vi "Get Calibration Data.vi"(0 "Base Path":path, 2 "Test Type":T1=1 items=["Practice Trials", "Mechanical (Mask)", "Mechanical (Mouthpiece)", "Labial (Normal)", "Labial (Quiet)", "Incomplete Interrupter", "Airflow Redirector", "Singing Helmet"], 5 "error in (no error)":errorcluster) -> (14 "Pressure Slope":dbl, 15 "Pressure Intercept":dbl, 16 "Microphone Sensitivity":dbl, 17 "SPL Gain":dbl, 18 "Flow Array":dbl[](array[numeric]), 19 "error out":errorcluster)   [LabVIEW 2020]
uses:
  Controls/Mech-Labial Test Types.ctl
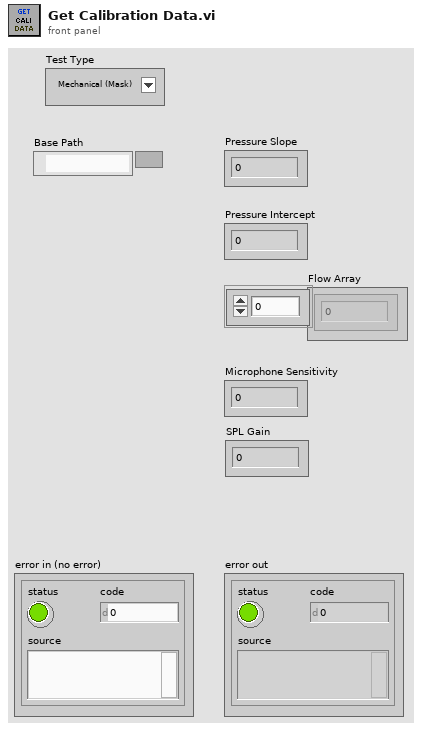
[diagram p1: front panel]
types:
  T1 = typedef "Mech-Labial Test Types.ctl" = u16
  T2 = enum16{"open", "replace", "create", "open or create", "replace or create", "replace or create with confirmation"}
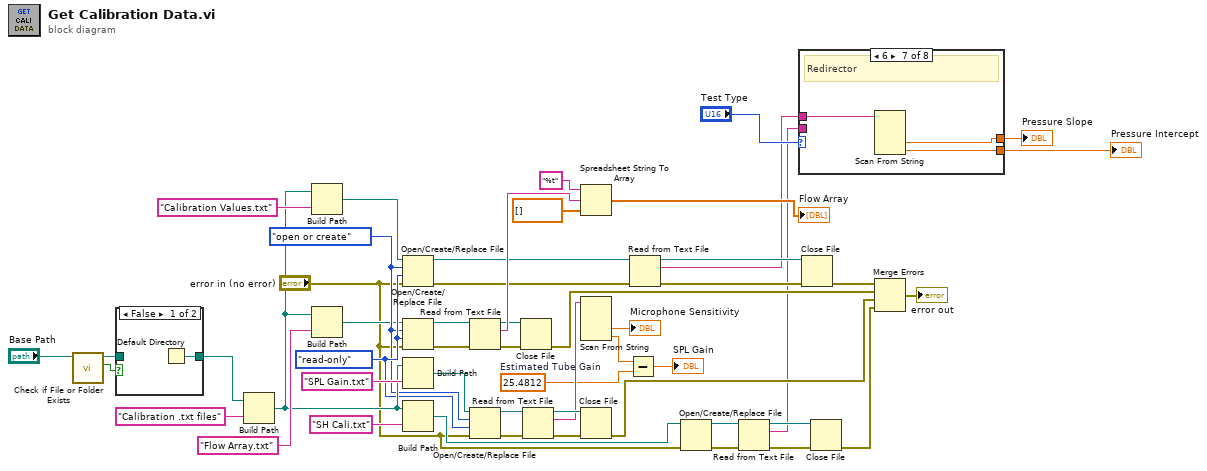
[diagram p0: block diagram]
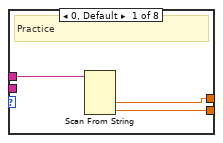
[diagram p2: hidden frame]
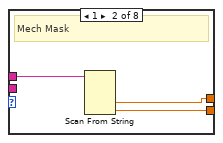
[diagram p3: hidden frame]
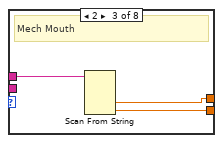
[diagram p4: hidden frame]
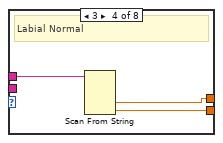
[diagram p5: hidden frame]
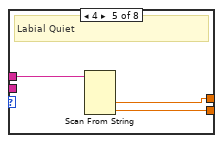
[diagram p6: hidden frame]
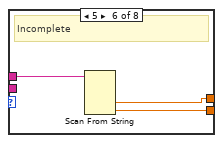
[diagram p7: hidden frame]
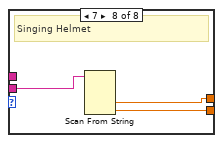
[diagram p8: hidden frame]
diagram:
  w6 = 25.4812  # Estimated Tube Gain
  w36 = enum16{"read/write", "read-only", "write-only"}."read-only" ("access (0:read/write)")
  w35 = T2."open or create" ("operation (0:open)")
  n1 = call <vilib>:"Check if File or Folder Exists.vi"("path"="Base Path") -> ("file or folder exists?"=w47:bool, "dup path"=w46:path)  [unwired: 8 in, 1 out]
  n2 = case shown="False" w47 {
    tunnel: w46 -> [_ w54]
    tunnel: [w53 w54] -> w45
    frame False {
      n3 = Default Directory() -> (w53:path)
    }
    frame True {
    }
  }
  n4 = Build Path(base path=w45, name or relative path="Calibration .txt files") -> (appended path=w44:path)
  n5 = Build Path(base path=w44, name or relative path="Calibration Values.txt") -> (appended path=w15:path)
  n6 = Build Path(base path=w44, name or relative path="Flow Array.txt") -> (appended path=w16:path)
  n7 = Open/Create/Replace File(file path (use dialog)=w15, error in="error in (no error)", operation (0:open)=w35, access (0:read/write)=w36) -> (refnum out=w19:refnum<file>, error out=w17:errorcluster)  [unwired: 2 in, 1 out]
  n8 = Open/Create/Replace File(file path (use dialog)=w16, error in="error in (no error)", operation (0:open)=w35, access (0:read/write)=w36) -> (refnum out=w23:refnum<file>, error out=w21:errorcluster)  [unwired: 2 in, 1 out]
  n9 = Build Path(base path=w44, name or relative path="SPL Gain.txt") -> (appended path=w14:path)
  n10 = Build Path(base path=w44, name or relative path="SH Cali.txt") -> (appended path=w13:path)
  n11 = Read from Text File(file (use dialog)=w23, error in=w21) -> (refnum out=w24:refnum<file>, text=w29:string, error out=w22:errorcluster)  [unwired: 2 in, 1 out]
  n12 = Open/Create/Replace File(file path (use dialog)=w14, error in="error in (no error)", operation (0:open)=w35, access (0:read/write)=w36) -> (refnum out=w32:refnum<file>, error out=w33:errorcluster)  [unwired: 2 in, 1 out]
  n13 = Close File(refnum=w24, error in=w22) -> (error out=w27:errorcluster)  [unwired: 1 out]
  n14 = Read from Text File(file (use dialog)=w32, error in=w33) -> (refnum out=w38:refnum<file>, text=w37:string, error out=w34:errorcluster)  [unwired: 2 in, 1 out]
  n15 = Spreadsheet String To Array(format string="%t", spreadsheet string=w29, array type (2D Dbl)=dbl[] []) -> (array=→"Flow Array":dbl[])  [unwired: 1 in]
  n16 = Scan From String(input string=w37) -> (output 1=→"Microphone Sensitivity":dbl, output 2=w41:dbl)  [unwired: 5 in, 3 out]
  n17 = Close File(refnum=w38, error in=w34) -> (error out=w39:errorcluster)  [unwired: 1 out]
  n18 = Subtract(x=w41, y=w6) -> (x-y=→"SPL Gain":dbl)
  n19 = Read from Text File(file (use dialog)=w19, error in=w17) -> (refnum out=w20:refnum<file>, text=w4:string, error out=w18:errorcluster)  [unwired: 2 in, 1 out]
  n20 = Open/Create/Replace File(file path (use dialog)=w13, error in="error in (no error)") -> (refnum out=w12:refnum<file>, error out=w10:errorcluster)  [unwired: 4 in, 1 out]
  n21 = Read from Text File(file (use dialog)=w12, error in=w10) -> (refnum out=w11:refnum<file>, text=w1:string, error out=w9:errorcluster)  [unwired: 2 in, 1 out]
  n22 = case shown="6" "Test Type" {
    tunnel: w4 -> [w57 w60 w63 w66 w69 w72 w73 _]
    tunnel: [w56 w59 w62 w65 w68 w71 w75 w77] -> w3
    tunnel: [w55 w58 w61 w64 w67 w70 w74 w76] -> w2
    tunnel: w1 -> [_ _ _ _ _ _ _ w78]
    frame 0, Default {
      # "Practice"
      n23 = Scan From String "Scan From String"(input string=w57) -> (output 1=w56:dbl, output 2=w55:dbl)  [unwired: 5 in, 3 out]
    }
    frame 1 {
      # "Mech Mask"
      n24 = Scan From String "Scan From String"(input string=w60) -> (output 1=w59:dbl, output 2=w58:dbl)  [unwired: 5 in, 3 out]
    }
    frame 2 {
      # "Mech Mouth"
      n25 = Scan From String "Scan From String"(input string=w63) -> (output 1=w62:dbl, output 2=w61:dbl)  [unwired: 5 in, 3 out]
    }
    frame 3 {
      # "Labial Normal"
      n26 = Scan From String "Scan From String"(input string=w66) -> (output 1=w65:dbl, output 2=w64:dbl)  [unwired: 5 in, 3 out]
    }
    frame 4 {
      # "Labial Quiet"
      n27 = Scan From String "Scan From String"(input string=w69) -> (output 1=w68:dbl, output 2=w67:dbl)  [unwired: 5 in, 3 out]
    }
    frame 5 {
      # "Incomplete"
      n28 = Scan From String "Scan From String"(input string=w72) -> (output 1=w71:dbl, output 2=w70:dbl)  [unwired: 5 in, 3 out]
    }
    frame 6 {
      # "Redirector"
      n29 = Scan From String "Scan From String"(input string=w73) -> (output 1=w75:dbl, output 2=w74:dbl)  [unwired: 5 in, 3 out]
    }
    frame 7 {
      # "Singing Helmet"
      n30 = Scan From String "Scan From String"(input string=w78) -> (output 1=w77:dbl, output 2=w76:dbl)  [unwired: 5 in, 3 out]
    }
  }
  "Pressure Intercept" <- w2
  "Pressure Slope" <- w3
  n31 = Close File(refnum=w20, error in=w18) -> (error out=w26:errorcluster)  [unwired: 1 out]
  n32 = Close File(refnum=w11, error in=w9) -> (error out=w8:errorcluster)  [unwired: 1 out]
  n33 = Merge Errors(w26, w27, w39, w8) -> (→"error out":errorcluster)
